vi "Set Last Name.vi"(8 "error in (no error)":errorcluster, 10 "Last Name":string, 11 "SOL User in":refnum<class "SOL User.lvclass">) -> (0 "error out":errorcluster, 3 "SOL User out":refnum<class "SOL User.lvclass">)   [LabVIEW 2020, in "Summer of LabVIEW.lvlib" / "SOL User.lvclass"]
uses:
  SOL User.lvclass
  SOL User.lvclass/SOL User.ctl
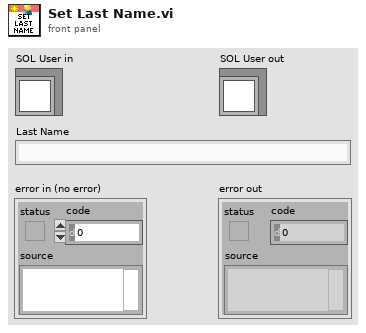
[diagram p1: front panel]
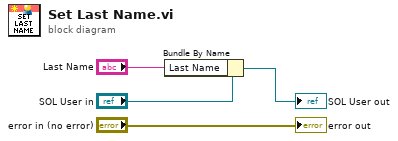
[diagram p0: block diagram]
diagram:
  n1 = Bundle By Name(cluster="SOL User in", "Last Name"="Last Name") -> (→"SOL User out":refnum<class "SOL User.lvclass">)
  "error out" <- "error in (no error)"
